vi "Lab Panel V4.86.vi"() -> ()   [LabVIEW 2013] (continued)
                          frame True {
                            n2237 = Bundle(cluster=w4041, "amps"=w4045, "volts"=w4044, "pf"=w4043) -> (w4042:cluster{"amps":dbl, "volts":dbl, "pf":dbl})
                            n2238 = local write "ON L05-1"(w4042) -> ()
                          }
                        }
                      }
                      frame #1 {
                        n2239 = Unbundle(w4050) -> ("amps"=w4049:dbl, "volts"=w4048:dbl, "pf"=w4047:dbl)
                        n2240 = case shown="True" w4051 {
                          tunnel: w4058 -> [_ w4090]
                          tunnel: w4057 -> [_ w4097]
                          tunnel: w4056 -> [_ _]
                          tunnel: w4055 -> [_ _]
                          tunnel: w4054 -> [_ w4096]
                          tunnel: w4053 -> [_ w4095]
                          tunnel: w4052 -> [_ w4060]
                          tunnel: w4049 -> [_ w4092]
                          tunnel: w4048 -> [_ w4091]
                          tunnel: w4047 -> [_ w4089]
                          tunnel: w4046 -> [_ w4081]
                          frame False {
                          }
                          frame True {
                            n2241 = local read "TDMS LAB05-1"() -> (w4094:refnum<k34>)
                            n2242 = Build Array(w4091) -> (w4086:dbl[])
                            n2243 = Build Array(w4089) -> (w4085:dbl[])
                            n2244 = Build Array(w4096) -> (w4084:dbl[])
                            n2245 = Build Array(w4097) -> (w4083:dbl[])
                            n2246 = Build Array(w4092) -> (w4088:dbl[])
                            n2247 = Build Array(w4090) -> (w4087:dbl[])
                            n2248 = Build Array(w4095) -> (w4082:dbl[])
                            n2249 = Build Array("AMPS ON", "AMPS OFF", "VOLTS", "PF", "TEMP Live", "TEMP Neut", "CYCLE") -> (w4065:string[])
                            n2250 = Bundle By Name("Y"=w4088, "t0"=w4081) -> (w4080:waveform(dbl))  [unwired: 1 in]
                            n2251 = Bundle By Name("Y"=w4087, "t0"=w4081) -> (w4079:waveform(dbl))  [unwired: 1 in]
                            n2252 = Bundle By Name("Y"=w4086, "t0"=w4081) -> (w4078:waveform(dbl))  [unwired: 1 in]
                            n2253 = Bundle By Name("Y"=w4085, "t0"=w4081) -> (w4077:waveform(dbl))  [unwired: 1 in]
                            n2254 = Bundle By Name("Y"=w4084, "t0"=w4081) -> (w4076:waveform(dbl))  [unwired: 1 in]
                            n2255 = Bundle By Name("Y"=w4083, "t0"=w4081) -> (w4075:waveform(dbl))  [unwired: 1 in]
                            n2256 = Bundle By Name("Y"=w4082, "t0"=w4081) -> (w4074:waveform(dbl))  [unwired: 1 in]
                            n2257 = Build Array(w4080, w4079, w4078, w4077, w4076, w4075, w4074) -> (w4073:waveform(dbl)[])
                            n2258 = TDMS Write(0:w4094, 5:"TEST VALUES", 7:w4065, 9:w4073) -> (4:w4064:refnum<k34>, 6:w4063:string, 15:w4062:errorcluster)  [unwired: 2 in, 1 out]
                            n2259 = TDMS Write(0:w4064, 5:w4063, 7:"TIME", 9:w4060, 11:w4062) -> (15:w4059:errorcluster)  [unwired: 1 in, 3 out]
                            n2260 = local write "data file error"(w4059) -> ()
                          }
                        }
                      }
                    }
                  }
                }
              }
              frame #9 {
                n2261 = case shown="True" w4098 {
                  tunnel: w4102 -> [_ w4107]
                  tunnel: w4101 -> [_ w4106]
                  tunnel: w4100 -> [_ w4104]
                  tunnel: w4099 -> [_ w4103]
                  frame False {
                  }
                  frame True {
                    n2262 = local read "DISP LAB05-2"() -> (w4108:T4)
                    n2263 = local read "SIG LAB05-2"() -> (w4109:T2)
                    n2264 = local read "ON L05-2"() -> (w4105:cluster{"amps":dbl, "volts":dbl, "pf":dbl})
                    n2265 = Unbundle(w4109) -> ("AMPS"=w4115:dbl, "VOLTS"=w4113:dbl, "PF"=w4112:dbl, "Tmp Live"=w4111:dbl, "Tmp Neut"=w4114:dbl)
                    n2266 = Unbundle(w4108) -> ("CYCLE"=w4110:dbl)  [unwired: 2 out]
                    n2267 = stacked-sequence {
                      tunnel: w4115 -> [w4119 w4138]
                      tunnel: w4114 -> [_ w4137]
                      tunnel: w4113 -> [w4118 w4136]
                      tunnel: w4112 -> [w4117 w4135]
                      tunnel: w4111 -> [_ w4134]
                      tunnel: w4110 -> [_ w4133]
                      tunnel: w4107 -> [_ w4132]
                      tunnel: w4106 -> [w4120 _]
                      tunnel: w4105 -> [w4116 w4130]
                      tunnel: w4104 -> [_ w4131]
                      tunnel: w4103 -> [_ w4126]
                      frame #0 {
                        n2268 = case shown="True" w4120 {
                          tunnel: w4119 -> [_ w4125]
                          tunnel: w4118 -> [_ w4124]
                          tunnel: w4117 -> [_ w4123]
                          tunnel: w4116 -> [_ w4121]
                          frame False {
                          }
                          frame True {
                            n2269 = Bundle(cluster=w4121, "amps"=w4125, "volts"=w4124, "pf"=w4123) -> (w4122:cluster{"amps":dbl, "volts":dbl, "pf":dbl})
                            n2270 = local write "ON L05-2"(w4122) -> ()
                          }
                        }
                      }
                      frame #1 {
                        n2271 = Unbundle(w4130) -> ("amps"=w4129:dbl, "volts"=w4128:dbl, "pf"=w4127:dbl)
                        n2272 = case shown="True" w4131 {
                          tunnel: w4138 -> [_ w4170]
                          tunnel: w4137 -> [_ w4177]
                          tunnel: w4136 -> [_ _]
                          tunnel: w4135 -> [_ _]
                          tunnel: w4134 -> [_ w4176]
                          tunnel: w4133 -> [_ w4175]
                          tunnel: w4132 -> [_ w4140]
                          tunnel: w4129 -> [_ w4172]
                          tunnel: w4128 -> [_ w4171]
                          tunnel: w4127 -> [_ w4169]
                          tunnel: w4126 -> [_ w4161]
                          frame False {
                          }
                          frame True {
                            n2273 = local read "TDMS LAB05-2"() -> (w4174:refnum<k34>)
                            n2274 = Build Array(w4171) -> (w4166:dbl[])
                            n2275 = Build Array(w4169) -> (w4165:dbl[])
                            n2276 = Build Array(w4176) -> (w4164:dbl[])
                            n2277 = Build Array(w4177) -> (w4163:dbl[])
                            n2278 = Build Array(w4172) -> (w4168:dbl[])
                            n2279 = Build Array(w4170) -> (w4167:dbl[])
                            n2280 = Build Array(w4175) -> (w4162:dbl[])
                            n2281 = Build Array("AMPS ON", "AMPS OFF", "VOLTS", "PF", "TEMP Live", "TEMP Neut", "CYCLE") -> (w4145:string[])
                            n2282 = Bundle By Name("Y"=w4168, "t0"=w4161) -> (w4160:waveform(dbl))  [unwired: 1 in]
                            n2283 = Bundle By Name("Y"=w4167, "t0"=w4161) -> (w4159:waveform(dbl))  [unwired: 1 in]
                            n2284 = Bundle By Name("Y"=w4166, "t0"=w4161) -> (w4158:waveform(dbl))  [unwired: 1 in]
                            n2285 = Bundle By Name("Y"=w4165, "t0"=w4161) -> (w4157:waveform(dbl))  [unwired: 1 in]
                            n2286 = Bundle By Name("Y"=w4164, "t0"=w4161) -> (w4156:waveform(dbl))  [unwired: 1 in]
                            n2287 = Bundle By Name("Y"=w4163, "t0"=w4161) -> (w4155:waveform(dbl))  [unwired: 1 in]
                            n2288 = Bundle By Name("Y"=w4162, "t0"=w4161) -> (w4154:waveform(dbl))  [unwired: 1 in]
                            n2289 = Build Array(w4160, w4159, w4158, w4157, w4156, w4155, w4154) -> (w4153:waveform(dbl)[])
                            n2290 = TDMS Write(0:w4174, 5:"TEST VALUES", 7:w4145, 9:w4153) -> (4:w4144:refnum<k34>, 6:w4143:string, 15:w4142:errorcluster)  [unwired: 2 in, 1 out]
                            n2291 = TDMS Write(0:w4144, 5:w4143, 7:"TIME", 9:w4140, 11:w4142) -> (15:w4139:errorcluster)  [unwired: 1 in, 3 out]
                            n2292 = local write "data file error"(w4139) -> ()
                          }
                        }
                      }
                    }
                  }
                }
              }
            }
          }
          frame #13 {
            # "display test values on chart"
            n2293 = disable-structure shown="Disabled" {
              frame Disabled {
                n2294 = case shown="\"ON CYCLE\", Default" w4186 {
                  tunnel: [1 _] -> _
                  frame "ON CYCLE", Default {
                  }
                  frame "OFF CYCLE" {
                  }
                }
              }
              frame Enabled {
              }
            }
            n2295 = local read "jig cycle"() -> (w4182:dbl)
            n2296 = local read "on loops"() -> (w4184:dbl)
            n2297 = Add(x=w4184, y=2) -> (x+y=w4181:dbl)
            n2298 = Equal?(x=w4182, y=1) -> (x = y?=w4180:bool)
            n2299 = Equal?(x=w4182, y=w4181) -> (x = y?=w4179:bool)
            n2300 = Or(x=w4180, y=w4179) -> (x .or. y?=w4178:bool)
            "graph flag" <- w4178
            n2301 = global write "Global display 3.vi" "graph flag"(w4178) -> ()
            n2302 = case shown="True" w4178 {
              frame False {
              }
              frame True {
                n2303 = local read "SIG LAB05-1"() -> (w4229:T2)
                n2304 = local read "SIG LAB04-2"() -> (w4230:T2)
                n2305 = local read "SIG LAB05-2"() -> (w4228:T2)
                n2306 = local read "SIG LAB04-1"() -> (w4231:T2)
                n2307 = local read "SIG LAB03-1"() -> (w4233:T2)
                n2308 = local read "SIG LAB03-2"() -> (w4232:T2)
                n2309 = local read "SIG LAB01-1"() -> (w4237:T2)
                n2310 = local read "SIG LAB02-2"() -> (w4234:T2)
                n2311 = local read "SIG LAB02-1"() -> (w4235:T2)
                n2312 = local read "SIG LAB01-2"() -> (w4236:T2)
                n2313 = Unbundle(w4230) -> ("AMPS"=w4220:dbl, "VOLTS"=w4210:dbl, "Tmp Live"=w4200:dbl, "Tmp Neut"=w4190:dbl)  [unwired: 1 out]
                n2314 = Unbundle(w4229) -> ("AMPS"=w4219:dbl, "VOLTS"=w4209:dbl, "Tmp Live"=w4199:dbl, "Tmp Neut"=w4189:dbl)  [unwired: 1 out]
                n2315 = Unbundle(w4228) -> ("AMPS"=w4218:dbl, "VOLTS"=w4208:dbl, "Tmp Live"=w4198:dbl, "Tmp Neut"=w4188:dbl)  [unwired: 1 out]
                n2316 = Unbundle(w4231) -> ("AMPS"=w4221:dbl, "VOLTS"=w4211:dbl, "Tmp Live"=w4201:dbl, "Tmp Neut"=w4191:dbl)  [unwired: 1 out]
                n2317 = Unbundle(w4232) -> ("AMPS"=w4222:dbl, "VOLTS"=w4212:dbl, "Tmp Live"=w4202:dbl, "Tmp Neut"=w4192:dbl)  [unwired: 1 out]
                n2318 = Unbundle(w4233) -> ("AMPS"=w4223:dbl, "VOLTS"=w4213:dbl, "Tmp Live"=w4203:dbl, "Tmp Neut"=w4193:dbl)  [unwired: 1 out]
                n2319 = Unbundle(w4234) -> ("AMPS"=w4224:dbl, "VOLTS"=w4214:dbl, "Tmp Live"=w4204:dbl, "Tmp Neut"=w4194:dbl)  [unwired: 1 out]
                n2320 = Unbundle(w4235) -> ("AMPS"=w4225:dbl, "VOLTS"=w4215:dbl, "Tmp Live"=w4205:dbl, "Tmp Neut"=w4195:dbl)  [unwired: 1 out]
                n2321 = Unbundle(w4237) -> ("AMPS"=w4227:dbl, "VOLTS"=w4217:dbl, "Tmp Live"=w4207:dbl, "Tmp Neut"=w4197:dbl)  [unwired: 1 out]
                n2322 = Unbundle(w4236) -> ("AMPS"=w4226:dbl, "VOLTS"=w4216:dbl, "Tmp Live"=w4206:dbl, "Tmp Neut"=w4196:dbl)  [unwired: 1 out]
                n2323 = stacked-sequence {
                  tunnel: w4227 -> [w4248 _ _ _ _]
                  tunnel: w4226 -> [w4247 _ _ _ _]
                  tunnel: w4225 -> [w4246 _ _ _ _]
                  tunnel: w4224 -> [w4245 _ _ _ _]
                  tunnel: w4223 -> [w4244 _ _ _ _]
                  tunnel: w4222 -> [w4243 _ _ _ _]
                  tunnel: w4221 -> [w4242 _ _ _ _]
                  tunnel: w4220 -> [w4241 _ _ _ _]
                  tunnel: w4219 -> [w4240 _ _ _ _]
                  tunnel: w4218 -> [w4239 _ _ _ _]
                  tunnel: w4217 -> [_ w4259 _ _ _]
                  tunnel: w4216 -> [_ w4258 _ _ _]
                  tunnel: w4215 -> [_ w4257 _ _ _]
                  tunnel: w4214 -> [_ w4256 _ _ _]
                  tunnel: w4213 -> [_ w4255 _ _ _]
                  tunnel: w4212 -> [_ w4254 _ _ _]
                  tunnel: w4211 -> [_ w4253 _ _ _]
                  tunnel: w4210 -> [_ w4252 _ _ _]
                  tunnel: w4209 -> [_ w4251 _ _ _]
                  tunnel: w4208 -> [_ w4250 _ _ _]
                  tunnel: w4207 -> [_ _ w4270 _ _]
                  tunnel: w4206 -> [_ _ w4269 _ _]
                  tunnel: w4205 -> [_ _ w4268 _ _]
                  tunnel: w4204 -> [_ _ w4267 _ _]
                  tunnel: w4203 -> [_ _ w4266 _ _]
                  tunnel: w4202 -> [_ _ w4265 _ _]
                  tunnel: w4201 -> [_ _ w4264 _ _]
                  tunnel: w4200 -> [_ _ w4263 _ _]
                  tunnel: w4199 -> [_ _ w4262 _ _]
                  tunnel: w4198 -> [_ _ w4261 _ _]
                  tunnel: w4197 -> [_ _ _ w4281 _]
                  tunnel: w4196 -> [_ _ _ w4280 _]
                  tunnel: w4195 -> [_ _ _ w4279 _]
                  tunnel: w4194 -> [_ _ _ w4278 _]
                  tunnel: w4193 -> [_ _ _ w4277 _]
                  tunnel: w4192 -> [_ _ _ w4276 _]
                  tunnel: w4191 -> [_ _ _ w4275 _]
                  tunnel: w4190 -> [_ _ _ w4274 _]
                  tunnel: w4189 -> [_ _ _ w4273 _]
                  tunnel: w4188 -> [_ _ _ w4272 _]
                  frame #0 {
                    n2324 = Merge Signals(w4248, w4247, w4246, w4245, w4244, w4243, w4242, w4241, w4240, w4239) -> (→"TEST AMPS CHART":dynamicdata)
                  }
                  frame #1 {
                    n2325 = Merge Signals(w4259, w4258, w4257, w4256, w4255, w4254, w4253, w4252, w4251, w4250) -> (→"TEST VOLTS CHART":dynamicdata)
                  }
                  frame #2 {
                    n2326 = Merge Signals(w4270, w4269, w4268, w4267, w4266, w4265, w4264, w4263, w4262, w4261) -> (→"TEMPERATURE (L) CHART":dynamicdata)
                  }
                  frame #3 {
                    n2327 = Merge Signals(w4281, w4280, w4279, w4278, w4277, w4276, w4275, w4274, w4273, w4272) -> (→"TEMPERATURE (N) CHART":dynamicdata)
                  }
                  frame #4 {
                    n2328 = local read "TEMPERATURE (N) CHART"() -> (w4282:dynamicdata)
                    n2329 = local read "TEMPERATURE (L) CHART"() -> (w4283:dynamicdata)
                    n2330 = local read "TEST VOLTS CHART"() -> (w4284:dynamicdata)
                    n2331 = local read "TEST AMPS CHART"() -> (w4285:dynamicdata)
                    n2332 = global write "Global display 3.vi" "graph temp N"(w4282) -> ()
                    n2333 = global write "Global display 3.vi" "graph temp L"(w4283) -> ()
                    n2334 = global write "Global display 3.vi" "graph volts"(w4284) -> ()
                    n2335 = global write "Global display 3.vi" "graph amps"(w4285) -> ()
                  }
                }
              }
            }
          }
          frame #14 {
            # "check for amps fail"
            # "check for cycle test & temperature rise fail conditions"
            n2336 = local read "on loops"() -> (w4312:dbl)
            n2337 = local read "jig cycle"() -> (w4309:dbl)
            n2338 = local read "jig cycle"() -> (w4314:dbl)
            n2339 = Add(x=w4312, y=3.0) -> (x+y=w4310:dbl)
            n2340 = Equal?(x=w4309, y=w4310) -> (x = y?=w4305:bool)
            n2341 = local read "Fail Loops"() -> (w4286:dbl)
            n2342 = Equal?(x=w4314, y=1.0) -> (x = y?=w4307:bool)
            n2343 = global write "Global 1.vi" "fail count"(w4286) -> ()
            n2344 = stacked-sequence {
              tunnel: w4308 -> [w4317 _ _ _ _ _ _ _ _ _]
              tunnel: w4307 -> [w4318 w4338 w4358 w4378 w4398 w4418 w4438 w4458 w4478 w4498]
              tunnel: w4306 -> [w4315 _ _ _ _ _ _ _ _ _]
              tunnel: w4305 -> [w4316 w4337 w4357 w4377 w4397 w4417 w4437 w4457 w4477 w4497]
              tunnel: w4304 -> [_ w4336 _ _ _ _ _ _ _ _]
              tunnel: w4303 -> [_ w4335 _ _ _ _ _ _ _ _]
              tunnel: w4302 -> [_ _ w4356 _ _ _ _ _ _ _]
              tunnel: w4301 -> [_ _ w4355 _ _ _ _ _ _ _]
              tunnel: w4300 -> [_ _ _ w4376 _ _ _ _ _ _]
              tunnel: w4299 -> [_ _ _ w4375 _ _ _ _ _ _]
              tunnel: w4298 -> [_ _ _ _ w4396 _ _ _ _ _]
              tunnel: w4297 -> [_ _ _ _ w4395 _ _ _ _ _]
              tunnel: w4296 -> [_ _ _ _ _ w4416 _ _ _ _]
              tunnel: w4295 -> [_ _ _ _ _ w4415 _ _ _ _]
              tunnel: w4294 -> [_ _ _ _ _ _ w4436 _ _ _]
              tunnel: w4293 -> [_ _ _ _ _ _ w4435 _ _ _]
              tunnel: w4292 -> [_ _ _ _ _ _ _ w4456 _ _]
              tunnel: w4291 -> [_ _ _ _ _ _ _ w4455 _ _]
              tunnel: w4290 -> [_ _ _ _ _ _ _ _ w4476 _]
              tunnel: w4289 -> [_ _ _ _ _ _ _ _ w4475 _]
              tunnel: w4288 -> [_ _ _ _ _ _ _ _ _ w4496]
              tunnel: w4287 -> [_ _ _ _ _ _ _ _ _ w4495]
              frame #0 {
                # "LAB01-1"
                n2345 = case shown="True" w4315 {
                  tunnel: w4318 -> [_ w4331]
                  tunnel: w4317 -> [_ w4328]
                  tunnel: w4316 -> [_ w4327]
                  frame False {
                  }
                  frame True {
                    n2346 = local read "TEMP START LAB01-1"() -> (w4333:cluster{"TL":dbl, "TN":dbl})
                    n2347 = local read "RESULT LAB01-1"() -> (w4322:bool)
                    n2348 = local read "FAIL LAB01-1"() -> (w4325:cluster{"LO":dbl, "HI":dbl})
                    n2349 = local read "TDMS LAB01-1"() -> (w4332:refnum<k34>)
                    n2350 = local read "SET LAB01-1"() -> (w4329:T5)
                    n2351 = local read "DISP LAB01-1"() -> (w4330:T4)
                    n2352 = local read "SIG LAB01-1"() -> (w4334:T2)
                    n2353 = Bundle("FAIL LAB01-1"=w4325, "SIG LAB01-1"=w4334, "TEMP START LAB01-1"=w4333, "DISP LAB01-1"=w4330, "SET LAB01-1"=w4329, "TDMS LAB01-1"=w4332) -> (w4319:T29)  [unwired: 1 in]
                    n2354 = call "sub vi - cycle&temp fail v6.vi"("Amps Lo?"=w4331, "Input Cluster"=w4319, "SELECT"=w4328, "Amps Hi?"=w4327, "Result In"=w4322) -> ("(FAIL) out"=w4324:cluster{"FAIL LO":dbl, "FAIL HI":dbl}, "(DISP) out"=w4320:T4, "T-RISE"=w4321:cluster{"T-RISE (L)":dbl, "T-RISE (N)":dbl}, "Result Out"=w4323:bool, "file error"=w4326:errorcluster)  [unwired: 10 in]
                    n2355 = local write "TEMP RISE LAB01-1"(w4321) -> ()
                    n2356 = local write "FAIL LAB01-1"(w4324) -> ()
                    n2357 = local write "DISP LAB01-1"(w4320) -> ()
                    n2358 = local write "RESULT LAB01-1"(w4323) -> ()
                    n2359 = local write "data file error"(w4326) -> ()
                  }
                }
              }
              frame #1 {
                # "LAB01-2"
                n2360 = case shown="True" w4336 {
                  tunnel: w4338 -> [_ w4351]
                  tunnel: w4335 -> [_ w4348]
                  tunnel: w4337 -> [_ w4347]
                  frame False {
                  }
                  frame True {
                    n2361 = local read "TEMP START LAB01-2"() -> (w4353:cluster{"TL":dbl, "TN":dbl})
                    n2362 = local read "FAIL LAB01-2"() -> (w4344:cluster{"LO":dbl, "HI":dbl})
                    n2363 = local read "TDMS LAB01-2"() -> (w4352:refnum<k34>)
                    n2364 = local read "SET LAB01-2"() -> (w4349:T5)
                    n2365 = local read "DISP LAB01-2"() -> (w4350:T4)
                    n2366 = local read "RESULT LAB01-2"() -> (w4341:bool)
                    n2367 = local read "SIG LAB01-2"() -> (w4354:T2)
                    n2368 = Bundle("FAIL LAB01-2"=w4344, "SIG LAB01-2"=w4354, "TEMP START LAB01-2"=w4353, "DISP LAB01-2"=w4350, "SET LAB01-2"=w4349, "TDMS LAB01-2"=w4352) -> (w4339:T30)  [unwired: 1 in]
                    n2369 = call "sub vi - cycle&temp fail v6.vi"("Amps Lo?"=w4351, "Input Cluster"=w4339, "SELECT"=w4348, "Amps Hi?"=w4347, "Result In"=w4341) -> ("(FAIL) out"=w4343:cluster{"FAIL LO":dbl, "FAIL HI":dbl}, "(DISP) out"=w4346:T4, "T-RISE"=w4340:cluster{"T-RISE (L)":dbl, "T-RISE (N)":dbl}, "Result Out"=w4342:bool, "file error"=w4345:errorcluster)  [unwired: 10 in]
                    n2370 = local write "TEMP RISE LAB01-2"(w4340) -> ()
                    n2371 = local write "FAIL LAB01-2"(w4343) -> ()
                    n2372 = local write "DISP LAB01-2"(w4346) -> ()
                    n2373 = local write "RESULT LAB01-2"(w4342) -> ()
                    n2374 = local write "data file error"(w4345) -> ()
                  }
                }
              }
              frame #2 {
                # "LAB02-1"
                n2375 = case shown="True" w4356 {
                  tunnel: w4358 -> [_ w4371]
                  tunnel: w4355 -> [_ w4368]
                  tunnel: w4357 -> [_ w4367]
                  frame False {
                  }
                  frame True {
                    n2376 = local read "TEMP START LAB02-1"() -> (w4373:cluster{"TL":dbl, "TN":dbl})
                    n2377 = local read "FAIL LAB02-1"() -> (w4364:cluster{"LO":dbl, "HI":dbl})
                    n2378 = local read "TDMS LAB02-1"() -> (w4372:refnum<k34>)
                    n2379 = local read "SET LAB02-1"() -> (w4369:T5)
                    n2380 = local read "DISP LAB02-1"() -> (w4370:T4)
                    n2381 = local read "SIG LAB02-1"() -> (w4374:T2)
                    n2382 = local read "RESULT LAB02-1"() -> (w4361:bool)
                    n2383 = Bundle("FAIL LAB02-1"=w4364, "SIG LAB02-1"=w4374, "TEMP START LAB02-1"=w4373, "DISP LAB02-1"=w4370, "SET LAB02-1"=w4369, "TDMS LAB02-1"=w4372) -> (w4359:T31)  [unwired: 1 in]
                    n2384 = call "sub vi - cycle&temp fail v6.vi"("Amps Lo?"=w4371, "Input Cluster"=w4359, "SELECT"=w4368, "Amps Hi?"=w4367, "Result In"=w4361) -> ("(FAIL) out"=w4363:cluster{"FAIL LO":dbl, "FAIL HI":dbl}, "(DISP) out"=w4366:T4, "T-RISE"=w4360:cluster{"T-RISE (L)":dbl, "T-RISE (N)":dbl}, "Result Out"=w4362:bool, "file error"=w4365:errorcluster)  [unwired: 10 in]
                    n2385 = local write "TEMP RISE LAB02-1"(w4360) -> ()
                    n2386 = local write "FAIL LAB02-1"(w4363) -> ()
                    n2387 = local write "DISP LAB02-1"(w4366) -> ()
                    n2388 = local write "RESULT LAB02-1"(w4362) -> ()
                    n2389 = local write "data file error"(w4365) -> ()
                  }
                }
              }
              frame #3 {
                # "LAB02-2"
                n2390 = case shown="True" w4376 {
                  tunnel: w4378 -> [_ w4391]
                  tunnel: w4375 -> [_ w4388]
                  tunnel: w4377 -> [_ w4387]
                  frame False {
                  }
                  frame True {
                    n2391 = local read "TEMP START LAB02-2"() -> (w4393:cluster{"TL":dbl, "TN":dbl})
                    n2392 = local read "FAIL LAB02-2"() -> (w4384:cluster{"LO":dbl, "HI":dbl})
                    n2393 = local read "TDMS LAB02-2"() -> (w4392:refnum<k34>)
                    n2394 = local read "SET LAB02-2"() -> (w4389:T5)
                    n2395 = local read "DISP LAB02-2"() -> (w4390:T4)
                    n2396 = local read "SIG LAB02-2"() -> (w4394:T2)
                    n2397 = local read "RESULT LAB02-2"() -> (w4381:bool)
                    n2398 = Bundle("FAIL LAB02-2"=w4384, "SIG LAB02-2"=w4394, "TEMP START LAB02-2"=w4393, "DISP LAB02-2"=w4390, "SET LAB02-2"=w4389, "TDMS LAB02-2"=w4392) -> (w4379:T32)  [unwired: 1 in]
                    n2399 = call "sub vi - cycle&temp fail v6.vi"("Amps Lo?"=w4391, "Input Cluster"=w4379, "SELECT"=w4388, "Amps Hi?"=w4387, "Result In"=w4381) -> ("(FAIL) out"=w4383:cluster{"FAIL LO":dbl, "FAIL HI":dbl}, "(DISP) out"=w4386:T4, "T-RISE"=w4380:cluster{"T-RISE (L)":dbl, "T-RISE (N)":dbl}, "Result Out"=w4382:bool, "file error"=w4385:errorcluster)  [unwired: 10 in]
                    n2400 = local write "TEMP RISE LAB02-2"(w4380) -> ()
                    n2401 = local write "FAIL LAB02-2"(w4383) -> ()
                    n2402 = local write "DISP LAB02-2"(w4386) -> ()
                    n2403 = local write "RESULT LAB02-2"(w4382) -> ()
                    n2404 = local write "data file error"(w4385) -> ()
                  }
                }
              }
              frame #4 {
                # "LAB03-1"
                n2405 = case shown="True" w4396 {
                  tunnel: w4398 -> [_ w4411]
                  tunnel: w4395 -> [_ w4408]
                  tunnel: w4397 -> [_ w4407]
                  frame False {
                  }
                  frame True {
                    n2406 = local read "TEMP START LAB03-1"() -> (w4413:cluster{"TL":dbl, "TN":dbl})
                    n2407 = local read "FAIL LAB03-1"() -> (w4404:cluster{"LO":dbl, "HI":dbl})
                    n2408 = local read "TDMS LAB03-1"() -> (w4412:refnum<k34>)
                    n2409 = local read "SET LAB03-1"() -> (w4409:T5)
                    n2410 = local read "DISP LAB03-1"() -> (w4410:T4)
                    n2411 = local read "SIG LAB03-1"() -> (w4414:T2)
                    n2412 = local read "RESULT LAB03-1"() -> (w4401:bool)
                    n2413 = Bundle("FAIL LAB03-1"=w4404, "SIG LAB03-1"=w4414, "TEMP START LAB03-1"=w4413, "DISP LAB03-1"=w4410, "SET LAB03-1"=w4409, "TDMS LAB03-1"=w4412) -> (w4399:T33)  [unwired: 1 in]
                    n2414 = call "sub vi - cycle&temp fail v6.vi"("Amps Lo?"=w4411, "Input Cluster"=w4399, "SELECT"=w4408, "Amps Hi?"=w4407, "Result In"=w4401) -> ("(FAIL) out"=w4403:cluster{"FAIL LO":dbl, "FAIL HI":dbl}, "(DISP) out"=w4406:T4, "T-RISE"=w4400:cluster{"T-RISE (L)":dbl, "T-RISE (N)":dbl}, "Result Out"=w4402:bool, "file error"=w4405:errorcluster)  [unwired: 10 in]
                    n2415 = local write "TEMP RISE LAB03-1"(w4400) -> ()
                    n2416 = local write "FAIL LAB03-1"(w4403) -> ()
                    n2417 = local write "DISP LAB03-1"(w4406) -> ()
                    n2418 = local write "RESULT LAB03-1"(w4402) -> ()
                    n2419 = local write "data file error"(w4405) -> ()
                  }
                }
              }
              frame #5 {
                # "LAB03-2"
                n2420 = case shown="True" w4416 {
                  tunnel: w4418 -> [_ w4431]
                  tunnel: w4415 -> [_ w4428]
                  tunnel: w4417 -> [_ w4427]
                  frame False {
                  }
                  frame True {
                    n2421 = local read "TEMP START LAB03-2"() -> (w4433:cluster{"TL":dbl, "TN":dbl})
                    n2422 = local read "FAIL LAB03-2"() -> (w4424:cluster{"LO":dbl, "HI":dbl})
                    n2423 = local read "TDMS LAB03-2"() -> (w4432:refnum<k34>)
                    n2424 = local read "SET LAB03-2"() -> (w4429:T5)
                    n2425 = local read "DISP LAB03-2"() -> (w4430:T4)
                    n2426 = local read "RESULT LAB03-2"() -> (w4421:bool)
                    n2427 = local read "SIG LAB03-2"() -> (w4434:T2)
                    n2428 = Bundle("FAIL LAB03-2"=w4424, "SIG LAB03-2"=w4434, "TEMP START LAB03-2"=w4433, "DISP LAB03-2"=w4430, "SET LAB03-2"=w4429, "TDMS LAB03-2"=w4432) -> (w4419:T34)  [unwired: 1 in]
                    n2429 = call "sub vi - cycle&temp fail v6.vi"("Amps Lo?"=w4431, "Input Cluster"=w4419, "SELECT"=w4428, "Amps Hi?"=w4427, "Result In"=w4421) -> ("(FAIL) out"=w4423:cluster{"FAIL LO":dbl, "FAIL HI":dbl}, "(DISP) out"=w4426:T4, "T-RISE"=w4420:cluster{"T-RISE (L)":dbl, "T-RISE (N)":dbl}, "Result Out"=w4422:bool, "file error"=w4425:errorcluster)  [unwired: 10 in]
                    n2430 = local write "FAIL LAB03-2"(w4423) -> ()
                    n2431 = local write "TEMP RISE LAB03-2"(w4420) -> ()
                    n2432 = local write "DISP LAB03-2"(w4426) -> ()
                    n2433 = local write "RESULT LAB03-2"(w4422) -> ()
                    n2434 = local write "data file error"(w4425) -> ()
                  }
                }
              }
              frame #6 {
                # "LAB04-1"
                n2435 = case shown="True" w4436 {
                  tunnel: w4438 -> [_ w4451]
                  tunnel: w4435 -> [_ w4448]
                  tunnel: w4437 -> [_ w4447]
                  frame False {
                  }
                  frame True {
                    n2436 = local read "TEMP START LAB04-1"() -> (w4453:cluster{"TL":dbl, "TN":dbl})
                    n2437 = local read "FAIL LAB04-1"() -> (w4444:cluster{"LO":dbl, "HI":dbl})
                    n2438 = local read "TDMS LAB04-1"() -> (w4452:refnum<k34>)
                    n2439 = local read "SET LAB04-1"() -> (w4449:T5)
                    n2440 = local read "DISP LAB04-1"() -> (w4450:T4)
                    n2441 = local read "SIG LAB04-1"() -> (w4454:T2)
                    n2442 = local read "RESULT LAB04-1"() -> (w4441:bool)
                    n2443 = Bundle("FAIL LAB04-1"=w4444, "SIG LAB04-1"=w4454, "TEMP START LAB04-1"=w4453, "DISP LAB04-1"=w4450, "SET LAB04-1"=w4449, "TDMS LAB04-1"=w4452) -> (w4439:T35)  [unwired: 1 in]
                    n2444 = call "sub vi - cycle&temp fail v6.vi"("Amps Lo?"=w4451, "Input Cluster"=w4439, "SELECT"=w4448, "Amps Hi?"=w4447, "Result In"=w4441) -> ("(FAIL) out"=w4443:cluster{"FAIL LO":dbl, "FAIL HI":dbl}, "(DISP) out"=w4446:T4, "T-RISE"=w4440:cluster{"T-RISE (L)":dbl, "T-RISE (N)":dbl}, "Result Out"=w4442:bool, "file error"=w4445:errorcluster)  [unwired: 10 in]
                    n2445 = local write "TEMP RISE LAB04-1"(w4440) -> ()
                    n2446 = local write "FAIL LAB04-1"(w4443) -> ()
                    n2447 = local write "DISP LAB04-1"(w4446) -> ()
                    n2448 = local write "RESULT LAB04-1"(w4442) -> ()
                    n2449 = local write "data file error"(w4445) -> ()
                  }
                }
              }
              frame #7 {
                # "LAB04-2"
                n2450 = case shown="True" w4456 {
                  tunnel: w4458 -> [_ w4471]
                  tunnel: w4455 -> [_ w4468]
                  tunnel: w4457 -> [_ w4467]
                  frame False {
                  }
                  frame True {
                    n2451 = local read "TEMP START LAB04-2"() -> (w4473:cluster{"TL":dbl, "TN":dbl})
                    n2452 = local read "FAIL LAB04-2"() -> (w4464:cluster{"LO":dbl, "HI":dbl})
                    n2453 = local read "TDMS LAB04-2"() -> (w4472:refnum<k34>)
                    n2454 = local read "SET LAB04-2"() -> (w4469:T5)
                    n2455 = local read "DISP LAB04-2"() -> (w4470:T4)
                    n2456 = local read "SIG LAB04-2"() -> (w4474:T2)
                    n2457 = local read "RESULT LAB04-2"() -> (w4461:bool)
                    n2458 = Bundle("FAIL LAB04-2"=w4464, "SIG LAB04-2"=w4474, "TEMP START LAB04-2"=w4473, "DISP LAB04-2"=w4470, "SET LAB04-2"=w4469, "TDMS LAB04-2"=w4472) -> (w4459:T36)  [unwired: 1 in]
                    n2459 = call "sub vi - cycle&temp fail v6.vi"("Amps Lo?"=w4471, "Input Cluster"=w4459, "SELECT"=w4468, "Amps Hi?"=w4467, "Result In"=w4461) -> ("(FAIL) out"=w4463:cluster{"FAIL LO":dbl, "FAIL HI":dbl}, "(DISP) out"=w4466:T4, "T-RISE"=w4460:cluster{"T-RISE (L)":dbl, "T-RISE (N)":dbl}, "Result Out"=w4462:bool, "file error"=w4465:errorcluster)  [unwired: 10 in]
                    n2460 = local write "TEMP RISE LAB04-2"(w4460) -> ()
                    n2461 = local write "FAIL LAB04-2"(w4463) -> ()
                    n2462 = local write "DISP LAB04-2"(w4466) -> ()
                    n2463 = local write "RESULT LAB04-2"(w4462) -> ()
                    n2464 = local write "data file error"(w4465) -> ()
                  }
                }
              }
              frame #8 {
                # "LAB05-1"
                n2465 = case shown="True" w4476 {
                  tunnel: w4478 -> [_ w4491]
                  tunnel: w4475 -> [_ w4488]
                  tunnel: w4477 -> [_ w4487]
                  frame False {
                  }
                  frame True {
                    n2466 = local read "TEMP START LAB05-1"() -> (w4493:cluster{"TL":dbl, "TN":dbl})
                    n2467 = local read "FAIL LAB05-1"() -> (w4484:cluster{"LO":dbl, "HI":dbl})
                    n2468 = local read "TDMS LAB05-1"() -> (w4492:refnum<k34>)
                    n2469 = local read "SET LAB05-1"() -> (w4489:T5)
                    n2470 = local read "DISP LAB05-1"() -> (w4490:T4)
                    n2471 = local read "SIG LAB05-1"() -> (w4494:T2)
                    n2472 = local read "RESULT LAB05-1"() -> (w4481:bool)
                    n2473 = Bundle("FAIL LAB05-1"=w4484, "SIG LAB05-1"=w4494, "TEMP START LAB05-1"=w4493, "DISP LAB05-1"=w4490, "SET LAB05-1"=w4489, "TDMS LAB05-1"=w4492) -> (w4479:T37)  [unwired: 1 in]
                    n2474 = call "sub vi - cycle&temp fail v6.vi"("Amps Lo?"=w4491, "Input Cluster"=w4479, "SELECT"=w4488, "Amps Hi?"=w4487, "Result In"=w4481) -> ("(FAIL) out"=w4483:cluster{"FAIL LO":dbl, "FAIL HI":dbl}, "(DISP) out"=w4486:T4, "T-RISE"=w4480:cluster{"T-RISE (L)":dbl, "T-RISE (N)":dbl}, "Result Out"=w4482:bool, "file error"=w4485:errorcluster)  [unwired: 10 in]
                    n2475 = local write "TEMP RISE LAB05-1"(w4480) -> ()
                    n2476 = local write "FAIL LAB05-1"(w4483) -> ()
                    n2477 = local write "DISP LAB05-1"(w4486) -> ()
                    n2478 = local write "RESULT LAB05-1"(w4482) -> ()
                    n2479 = local write "data file error"(w4485) -> ()
                  }
                }
              }
              frame #9 {
                # "LAB05-2"
                n2480 = case shown="True" w4496 {
                  tunnel: w4498 -> [_ w4511]
                  tunnel: w4495 -> [_ w4508]
                  tunnel: w4497 -> [_ w4507]
                  frame False {
                  }
                  frame True {
                    n2481 = local read "TEMP START LAB05-2"() -> (w4513:cluster{"TL":dbl, "TN":dbl})
                    n2482 = local read "FAIL LAB05-2"() -> (w4504:cluster{"LO":dbl, "HI":dbl})
                    n2483 = local read "TDMS LAB05-2"() -> (w4512:refnum<k34>)
                    n2484 = local read "SET LAB05-2"() -> (w4509:T5)
                    n2485 = local read "DISP LAB05-2"() -> (w4510:T4)
                    n2486 = local read "SIG LAB05-2"() -> (w4514:T2)
                    n2487 = local read "RESULT LAB05-2"() -> (w4501:bool)
                    n2488 = Bundle("FAIL LAB05-2"=w4504, "SIG LAB05-2"=w4514, "TEMP START LAB05-2"=w4513, "DISP LAB05-2"=w4510, "SET LAB05-2"=w4509, "TDMS LAB05-2"=w4512) -> (w4499:T38)  [unwired: 1 in]
                    n2489 = call "sub vi - cycle&temp fail v6.vi"("Amps Lo?"=w4511, "Input Cluster"=w4499, "SELECT"=w4508, "Amps Hi?"=w4507, "Result In"=w4501) -> ("(FAIL) out"=w4503:cluster{"FAIL LO":dbl, "FAIL HI":dbl}, "(DISP) out"=w4506:T4, "T-RISE"=w4500:cluster{"T-RISE (L)":dbl, "T-RISE (N)":dbl}, "Result Out"=w4502:bool, "file error"=w4505:errorcluster)  [unwired: 10 in]
                    n2490 = local write "TEMP RISE LAB05-2"(w4500) -> ()
                    n2491 = local write "FAIL LAB05-2"(w4503) -> ()
                    n2492 = local write "DISP LAB05-2"(w4506) -> ()
                    n2493 = local write "RESULT LAB05-2"(w4502) -> ()
                    n2494 = local write "data file error"(w4505) -> ()
                  }
                }
              }
            }
          }
          frame #15 {
            # "run calibration routine"
            n2495 = local read "SET (cal)"() -> (w4515:bool)
            n2496 = case shown="True" w4515 {
              frame False {
              }
              frame True {
                n2497 = stacked-sequence {
                  seq-local: [w4516 _ _] -> [_ w4518 _]
                  frame #0 {
                    n2498 = call "CALIBRATION PASSWORD"() -> ("PASSWORD"=w4516:string)  [unwired: 17 in, 2 out]
                  }
                  frame #1 {
                    n2499 = Equal?(x=w4518, y="7777") -> (x = y?=w4517:bool)
                    n2500 = case shown="True" w4517 {
                      frame False {
                      }
                      frame True {
                        n2501 = stacked-sequence {
                          frame #0 {
                            n2502 = call "sub vi - calibration v1.vi"() -> ()  [unwired: 12 in]
                          }
                          frame #1 {
                            n2503 = call "sub vi - get calibration values v1.vi"() -> ("LAB01 (CAL)"=w4524:T12, "LAB02 (CAL)"=w4523:T13, "LAB03 (CAL)"=w4522:T12, "LAB04 (CAL)"=w4521:T12, "calibration file error out"=w4525:errorcluster, "LAB05 (CAL)"=w4520:T12)  [unwired: 9 in, 1 out]
                            n2504 = local write "cal file error out"(w4525) -> ()
                            n2505 = local write "CAL LAB04"(w4521) -> ()
                            n2506 = local write "CAL LAB05"(w4520) -> ()
                            n2507 = local write "CAL LAB01"(w4524) -> ()
                            n2508 = local write "CAL LAB02"(w4523) -> ()
                            n2509 = local write "CAL LAB03"(w4522) -> ()
                          }
                        }
                      }
                    }
                  }
                  frame #2 {
                    n2510 = local write "SET (cal)"(FALSE) -> ()
                  }
                }
              }
            }
          }
          frame #16 {
            # "save certain settings to file"
            n2511 = String To Path(string="c:\\crabtree\\Set Up\\") -> (path=w4528:path)
            n2512 = Build Path(base path=w4528, name or relative path="settings.bin") -> (appended path=w4530:path)
            n2513 = Build Path(base path=w4528, name or relative path="mail.bin") -> (appended path=w4527:path)
            n2514 = Create Folder(path (use dialog)=w4528) -> (error out=w4533:errorcluster)  [unwired: 2 in, 2 out]
            n2515 = call <vilib>:"Clear Errors.vi"("error in (no error)"=w4533) -> ()  [unwired: 6 in, 1 out]
            n2516 = stacked-sequence {
              seq-local: [w4545 _] -> [_ w4558]
              tunnel: w4530 -> [_ w4559]
              tunnel: w4527 -> [_ w4557]
              frame #0 {
                n2517 = local read "C drive data root dir"() -> (w4544:path)
                n2518 = local read "Select COM port"() -> (w4541:refnum<visa-resource-name>)
                n2519 = local read "Network Directory"() -> (w4550:path)
                n2520 = local read "SET LAB05-2"() -> (w4549:T5)
                n2521 = local read "SET LAB05-1"() -> (w4548:T5)
                n2522 = local read "SET LAB04-2"() -> (w4547:T5)
                n2523 = local read "SET LAB03-2"() -> (w4551:T5)
                n2524 = local read "SET LAB04-1"() -> (w4546:T5)
                n2525 = local read "SET LAB03-1"() -> (w4552:T5)
                n2526 = local read "SET LAB02-2"() -> (w4553:T5)
                n2527 = local read "SET LAB02-1"() -> (w4554:T5)
                n2528 = local read "Temp Delay Lps"() -> (w4540:dbl)
                n2529 = local read "SET LAB01-2"() -> (w4555:T5)
                n2530 = local read "Temp Test Cal"() -> (w4537:dbl)
                n2531 = local read "SET LAB01-1"() -> (w4556:T5)
                n2532 = local read "Mail Test File To:"() -> (w4535:string)
                n2533 = local read "Temp Value"() -> (w4539:dbl)
                n2534 = local read "Fail Loops"() -> (w4538:dbl)
                n2535 = local read "spare"() -> (w4536:dbl)
                n2536 = local read "Mail Test Fail"() -> (w4534:bool)
                n2537 = local read "RATE (Hz)"() -> (w4543:dbl)
                n2538 = local read "SAMPLES"() -> (w4542:dbl)
                n2539 = Bundle("SET LAB01-1"=w4556, "SET LAB01-2"=w4555, "SET LAB02-1"=w4554, "SET LAB02-2"=w4553, "SET LAB03-1"=w4552, "SET LAB03-2"=w4551, "SET LAB04-1"=w4546, "SET LAB04-2"=w4547, "SET LAB05-1"=w4548, "SET LAB05-2"=w4549, "Network Directory"=w4550, "C drive data root dir"=w4544, "RATE (Hz)"=w4543, "SAMPLES"=w4542, "Select COM port"=w4541, "Temp Delay Lps"=w4540, "Temp Value"=w4539, "Fail Loops"=w4538, "Temp Test Cal"=w4537, "spare"=w4536, "Mail Test File To:"=w4535, "Mail Test Fail"=w4534) -> (w4545:T20)  [unwired: 1 in]
              }
              frame #1 {
                n2540 = event shown="[1] \"SET LAB01-1\", \"SET LAB01-2\", \"SET LAB02-1\", \"SET LAB02-2\", \"SET LAB03-1\", \"SET LAB03-2\", \"SET LAB04-1\", \"SET LAB04-2\", \"SET LAB05-1\", \"SET LAB05-2\", \"Network Directory\", \"C drive data root dir\", \"RATE (Hz)\", \"SAMPLES\", \"Select COM port\", \"Temp Delay Lps\", \"Temp Value\", \"Fail Loops\", \"Temp Test Cal\", \"spare\", \"Mail Test File To:\", \"Mail Test Fail\": Value Change" {
                  selector: _ -> [_ _ _]
                  dyn-events: _ -> [_ _ _]
                  timeout: 10.0 -> [_ _ _]
                  tunnel: w4559 -> [_ w4561 _]
                  tunnel: w4558 -> [_ w4562 _]
                  tunnel: w4557 -> [_ _ w4573]
                  event Timeout {
                    n2541 = event-data() -> ()  [unwired: 1 in, 3 out]
                  }
                  event "SET LAB01-1", "SET LAB01-2", "SET LAB02-1", "SET LAB02-2", "SET LAB03-1", "SET LAB03-2", "SET LAB04-1", "SET LAB04-2", "SET LAB05-1", "SET LAB05-2", "Network Directory", "C drive data root dir", "RATE (Hz)", "SAMPLES", "Select COM port", "Temp Delay Lps", "Temp Value", "Fail Loops", "Temp Test Cal", "spare", "Mail Test File To:", "Mail Test Fail": Value Change {
                    n2542 = event-data() -> ()  [unwired: 1 in, 6 out]
                    n2543 = Open/Create/Replace File(file path (use dialog)=w4561, operation (0:open)=T19."replace or create") -> (refnum out=w4567:refnum<file>, error out=w4566:errorcluster)  [unwired: 4 in, 1 out]
                    n2544 = Write to Binary File(file (use dialog)=w4567, data=w4562, error in=w4566) -> (refnum out=w4565:refnum<file>, error out=w4564:errorcluster)  [unwired: 3 in, 1 out]
                    n2545 = Close File(refnum=w4565, error in=w4564) -> (error out=w4563:errorcluster)  [unwired: 1 out]
                    n2546 = local write "data file error"(w4563) -> ()
                  }
                  event "MAIL SETTINGS.OUT SERVER ADDRESS", "MAIL SETTINGS.FROM ACCOUNT", "MAIL SETTINGS.USER NAME", "MAIL SETTINGS.PASSWORD", "Auto Mail Send", "TO (string):": Value Change {
                    n2547 = event-data() -> ()  [unwired: 1 in, 6 out]
                    n2548 = local read "MAIL SETTINGS"() -> (w4572:T6)
                    n2549 = local read "Auto Mail Send"() -> (w4570:bool)
                    n2550 = local read "TO (string):"() -> (w4569:string)
                    n2551 = Open/Create/Replace File(file path (use dialog)=w4573, operation (0:open)=T19."replace or create") -> (refnum out=w4578:refnum<file>, error out=w4577:errorcluster)  [unwired: 4 in, 1 out]
                    n2552 = Bundle("MAIL SETTINGS"=w4572, "Auto Mail Send"=w4570, "TO (string):"=w4569) -> (w4571:T39)  [unwired: 1 in]
                    n2553 = Write to Binary File(file (use dialog)=w4578, data=w4571, error in=w4577) -> (refnum out=w4576:refnum<file>, error out=w4575:errorcluster)  [unwired: 3 in, 1 out]
                    n2554 = Close File(refnum=w4576, error in=w4575) -> (error out=w4574:errorcluster)  [unwired: 1 out]
                    n2555 = local write "data file error"(w4574) -> ()
                  }
                }
              }
            }
          }
          frame #17 {
            # "mail control"
            n2556 = local read "MAIL SETTINGS"() -> (w4595:T6)
            n2557 = local read "Auto Mail Send"() -> (w4581:bool)
            n2558 = Unbundle(w4595) -> ("OUT SERVER ADDRESS"=w4594:string, "FROM ACCOUNT"=w4593:string, "TEST MAIL"=w4592:bool)  [unwired: 4 out]
            n2559 = stacked-sequence {
              tunnel: "TO (string):" -> [_ w4634]
              tunnel: w4595 -> [w4600 w4633]
              tunnel: w4594 -> [w4599 w4632]
              tunnel: w4593 -> [w4598 w4631]
              tunnel: w4592 -> [w4597 _]
              tunnel: w4581 -> [_ w4630]
              tunnel: w4591 -> [_ w4629]
              tunnel: w4590 -> [_ w4628]
              tunnel: w4589 -> [_ w4627]
              tunnel: w4588 -> [_ w4626]
              tunnel: w4587 -> [_ w4625]
              tunnel: w4586 -> [_ w4624]
              tunnel: w4585 -> [_ w4623]
              tunnel: w4584 -> [_ w4622]
              tunnel: w4583 -> [_ w4621]
              tunnel: w4582 -> [_ w4620]
              tunnel: "TO (string):" -> [w4596 _]
              frame #0 {
                # "mail test"
                n2560 = case shown="True" w4597 {
                  tunnel: w4600 -> [_ w4604]
                  tunnel: w4596 -> [_ w4603]
                  tunnel: w4599 -> [_ w4602]
                  tunnel: w4598 -> [_ w4601]
                  frame False {
                  }
                  frame True {
                    n2561 = stacked-sequence {
                      seq-local: [_ _ w4614 _] -> [_ _ _ w4615]
                      tunnel: w4604 -> [w4607 _ _ w4619]
                      tunnel: w4603 -> [_ _ w4612 _]
                      tunnel: w4602 -> [_ _ w4610 _]
                      tunnel: w4601 -> [_ _ w4611 _]
                      frame #0 {
                        n2562 = Bundle(cluster=w4607, "TEST MAIL STATUS"="TEST START") -> (w4605:T6)  [unwired: 6 in]
                        n2563 = local write "MAIL SETTINGS"(w4605) -> ()
                      }
                      frame #1 {
                        n2564 = Wait (ms)(milliseconds to wait=500) -> ()  [unwired: 1 out]
                      }
                      frame #2 {
                        n2565 = call "sub vi - send mail v5.vi"("TO:"=w4612, "subject"="MAIL TEST FROM LAB PANEL", "from"=w4611, "out going server"=w4610, "message"="TEST MESSAGE") -> ("error out"=w4614:errorcluster)  [unwired: 10 in]
                      }
                      frame #3 {
                        n2566 = Bundle(cluster=w4619, "TEST MAIL"=FALSE, "TEST MAIL STATUS"="TEST END", "mail error"=w4615) -> (w4617:T6)  [unwired: 4 in]
                        n2567 = local write "MAIL SETTINGS"(w4617) -> ()
                      }
                    }
                  }
                }
              }
              frame #1 {
                # "mail report"
                n2568 = stacked-sequence {
                  seq-local: [_ w4677 _ _] -> [_ _ _ w4867]
                  seq-local: [_ _ w4780 _] -> [_ _ _ w4857]
                  seq-local: [w4644 _ _ _] -> [_ w4694 _ _]
                  seq-local: [w4643 _ _ _] -> [_ w4693 _ _]
                  seq-local: [w4641 _ _ _] -> [_ w4691 _ _]
                  seq-local: [w4642 _ _ _] -> [_ w4692 _ _]
                  seq-local: [w4640 _ _ _] -> [_ w4690 _ _]
                  seq-local: [w4639 _ _ _] -> [_ w4685 _ _]
                  seq-local: [w4638 _ _ _] -> [_ w4686 _ _]
                  seq-local: [w4637 _ _ _] -> [_ w4687 _ _]
                  seq-local: [w4636 _ _ _] -> [_ w4688 _ _]
                  seq-local: [w4635 _ _ _] -> [_ w4689 _ _]
                  tunnel: w4634 -> [_ _ _ w4868]
                  tunnel: w4633 -> [_ _ _ w4851]
                  tunnel: w4632 -> [_ _ _ w4865]
                  tunnel: w4631 -> [_ _ _ w4864]
                  tunnel: w4630 -> [w4675 _ _ w4859]
                  tunnel: w4629 -> [_ _ w4810 _]
                  tunnel: w4628 -> [_ _ w4807 _]
                  tunnel: w4627 -> [_ _ w4806 _]
                  tunnel: w4626 -> [_ _ w4805 _]
                  tunnel: w4625 -> [_ _ w4804 _]
                  tunnel: w4624 -> [_ _ w4803 _]
                  tunnel: w4623 -> [_ _ w4802 _]
                  tunnel: w4622 -> [_ _ w4801 _]
                  tunnel: w4621 -> [_ _ w4800 _]
                  tunnel: w4620 -> [_ _ w4799 _]
                  frame #0 {
                    n2569 = case shown="False" w4675 {
                      frame False {
                        n2570 = local write "mail control"("") -> ()
                      }
                      frame True {
                      }
                    }
                    n2571 = local read "SET LAB01-1"() -> (w4674:T5)
                    n2572 = local read "SET LAB01-2"() -> (w4673:T5)
                    n2573 = local read "SET LAB02-1"() -> (w4672:T5)
                    n2574 = local read "SET LAB02-2"() -> (w4671:T5)
                    n2575 = local read "SET LAB03-1"() -> (w4670:T5)
                    n2576 = local read "SET LAB04-1"() -> (w4668:T5)
                    n2577 = local read "SET LAB05-1"() -> (w4666:T5)
                    n2578 = local read "SET LAB03-2"() -> (w4669:T5)
                    n2579 = local read "SET LAB04-2"() -> (w4667:T5)
                    n2580 = local read "SET LAB05-2"() -> (w4665:T5)
